vi "CRD CVT2.vi"(8 "error in":errorcluster, 11 "Controller in":refnum<class "Controller.lvclass">) -> (0 "error out":errorcluster, 3 "Controller out":refnum<class "Controller.lvclass">)   [LabVIEW 2014]
uses:
  <vilib>/Utility/config.llb/NI_LVConfig.lvlib
  <vilib>/Utility/config.llb/Read Key (String).vi
  <vilib>/Utility/config.llb/Read Key (Double).vi
  Controller.lvclass
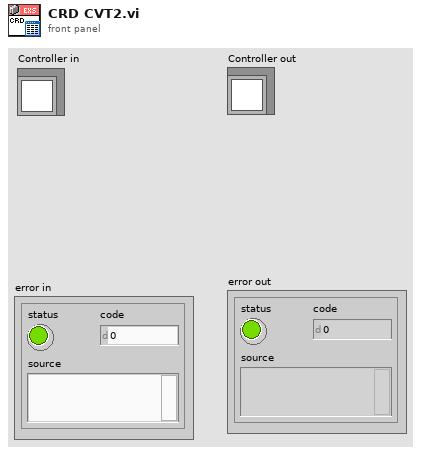
[diagram p1: front panel]
types:
  T1 = typedef "NI_LVConfig.lvlib/Config Data RefNum.ctl" = refnum<k1>
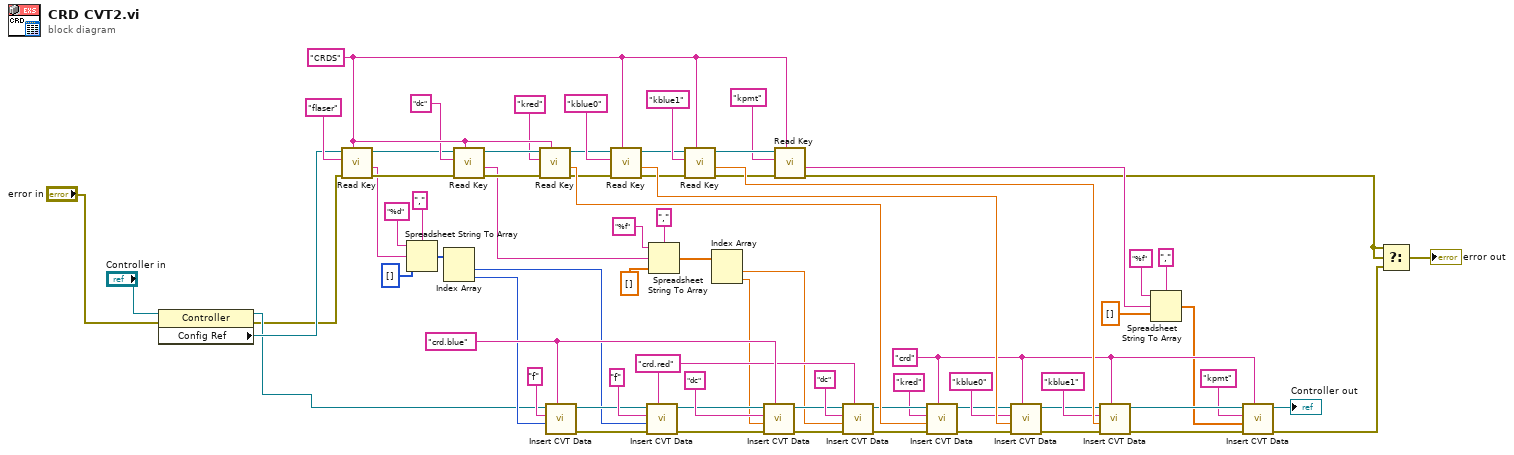
[diagram p0: block diagram]
diagram:
  w73 = "crd.blue" ("Group")
  w72 = "crd.red" ("Group")
  w62 = "crd" ("Group")
  w55 = "CRDS" ("section")
  n1 = property class="Controller"(reference="Controller in", error in="error in") -> (reference out=w3:refnum<class "Controller.lvclass">, error out=w1:errorcluster, "Config Ref"=w5:T1)
  n2 = call-poly <vilib>:"Read Key.vi"("section"=w55, "error in (no error)"=w1, "key"="flaser", "refnum"=w5) -> ("error out"=w35:errorcluster, "value"=w17:string, "refnum out"=w34:T1)  [unwired: 4 in, 1 out]
  n3 = Spreadsheet String To Array(delimiter (Tab)=",", format string="%d", spreadsheet string=w17, array type (2D Dbl)=i16[] []) -> (array=w20:i16[])
  n4 = Index Array(array=w20) -> (element #1=w12:i16, element #2=w13:i16)  [unwired: 2 in]
  n5 = call-poly <vilib>:"Read Key.vi"("section"=w55, "error in (no error)"=w35, "key"="dc", "refnum"=w34) -> ("error out"=w41:errorcluster, "value"=w39:string, "refnum out"=w40:T1)  [unwired: 4 in, 1 out]
  n6 = call-poly <vilib>:"Read Key.vi"("section"=w55, "error in (no error)"=w41, "key"="kred" ("section"), "refnum"=w40) -> ("error out"=w52:errorcluster, "value"=w60:dbl, "refnum out"=w51:T1)  [unwired: 4 in, 1 out]
  n7 = call "Insert CVT Data.vi"("Group"=w73, "Data"=w13, "tag"="f" ("Tag Name"), "Controller in"=w3) -> ("error out"=w31:errorcluster, "Controller out"=w26:refnum<class "Controller.lvclass">)  [unwired: 6 in]
  n8 = call-poly <vilib>:"Read Key.vi"("section"=w55, "error in (no error)"=w52, "key"="kblue0", "refnum"=w51) -> ("error out"=w54:errorcluster, "value"=w70:dbl, "refnum out"=w53:T1)  [unwired: 4 in, 1 out]
  n9 = call "Insert CVT Data.vi"("Group"=w72, "error in"=w31, "Data"=w12, "tag"="f" ("Tag Name"), "Controller in"=w26) -> ("error out"=w46:errorcluster, "Controller out"=w42:refnum<class "Controller.lvclass">)  [unwired: 5 in]
  n10 = Spreadsheet String To Array(delimiter (Tab)=",", format string="%f", spreadsheet string=w39, array type (2D Dbl)=sgl[] []) -> (array=w50:sgl[])
  n11 = call-poly <vilib>:"Read Key.vi"("section"=w55, "error in (no error)"=w54, "key"="kblue1", "refnum"=w53) -> ("error out"=w57:errorcluster, "value"=w71:dbl, "refnum out"=w56:T1)  [unwired: 4 in, 1 out]
  n12 = Index Array(array=w50) -> (element #1=w10:sgl, element #2=w11:sgl)  [unwired: 2 in]
  n13 = call "Insert CVT Data.vi"("Group"=w73, "error in"=w46, "Data"=w11, "tag"="dc", "Controller in"=w42) -> ("error out"=w45:errorcluster, "Controller out"=w43:refnum<class "Controller.lvclass">)  [unwired: 5 in]
  n14 = call-poly <vilib>:"Read Key.vi"("section"=w55, "error in (no error)"=w57, "key"="kpmt" ("section"), "refnum"=w56) -> ("error out"=w7:errorcluster, "value"=w22:string)  [unwired: 4 in, 2 out]
  n15 = call "Insert CVT Data.vi"("Group"=w72, "error in"=w45, "Data"=w10, "tag"="dc", "Controller in"=w43) -> ("error out"=w47:errorcluster, "Controller out"=w44:refnum<class "Controller.lvclass">)  [unwired: 5 in]
  n16 = call "Insert CVT Data.vi"("Group"=w62, "error in"=w47, "Data"=w60, "tag"="kred" ("Tag Name"), "Controller in"=w44) -> ("error out"=w65:errorcluster, "Controller out"=w61:refnum<class "Controller.lvclass">)  [unwired: 5 in]
  n17 = call "Insert CVT Data.vi"("Group"=w62, "error in"=w65, "Data"=w70, "tag"="kblue0", "Controller in"=w61) -> ("error out"=w66:errorcluster, "Controller out"=w63:refnum<class "Controller.lvclass">)  [unwired: 5 in]
  n18 = call "Insert CVT Data.vi"("Group"=w62, "error in"=w66, "Data"=w71, "tag"="kblue1", "Controller in"=w63) -> ("error out"=w67:errorcluster, "Controller out"=w64:refnum<class "Controller.lvclass">)  [unwired: 5 in]
  n19 = Spreadsheet String To Array(delimiter (Tab)=",", format string="%f", spreadsheet string=w22, array type (2D Dbl)=sgl[] []) -> (array=w29:sgl[])
  n20 = call "Insert CVT Data.vi"("Group"=w62, "error in"=w67, "Data"=w29, "tag"="kpmt" ("Tag Name"), "Controller in"=w64) -> ("error out"=w8:errorcluster, "Controller out"=→"Controller out":refnum<class "Controller.lvclass">)  [unwired: 5 in]
  n21 = Select(t=w7, s=w7, f=w8) -> (s? t:f=→"error out":errorcluster)
